vi "rs3 get api version.vi"(8 "error in (no error)":errorcluster) -> (0 "error out":errorcluster, 3 "version":i32=20000)   [LabVIEW 2017, in "libRealSense3.lvlib"]
doc: "This retrieves the version number of the libRealSense library. \nThe output needs to be passed to Create Device."
uses:
  <vilib>/addons/RealSense/libRealSense3.lvlib
  <vilib>/addons/RealSense/realsense-d.dll
panel:
  # "RS2 Get API Version"
  # "(C) Intel Corp.,  AGJ"
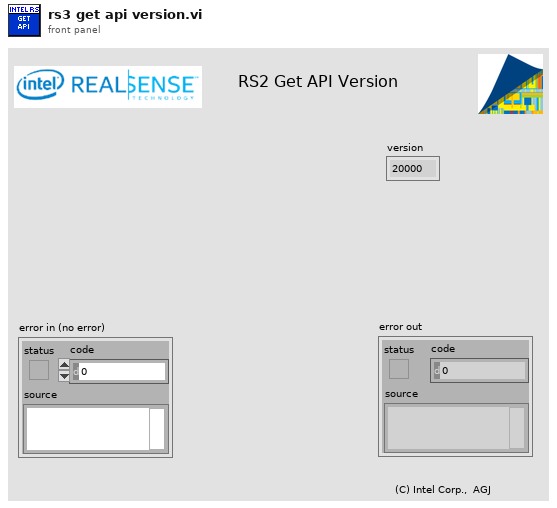
[diagram p1: front panel]
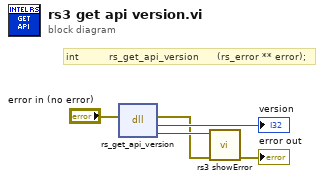
[diagram p0: block diagram]
diagram:
  # "int          rs_get_api_version      (rs_error ** error);"
  n1 = dll-call lib="C:/Program Files (x86)/National Instruments/LabVIEW 2017/vi.lib/addons/RealSense/realsense-d.dll" fn="rs_get_api_version"(error in="error in (no error)") -> (error out=w2:errorcluster, "return type"=→"version":i32, "error"=w3:u64)  [unwired: 3 in, 1 out]
  n2 = call <vilib>:"rs3 showError.vi"("error in (no error)"=w2, "error"=w3) -> ("error out"=→"error out":errorcluster)  [unwired: 5 in, 4 out]
